vi "Event to CSV String PyExcel.vi"(8 "error in (no error)":errorcluster, 11 "Event":T1) -> (0 "error out":errorcluster, 2 "String":string)   [LabVIEW 2019, in "Logger.lvlib" / "Logger.lvclass"]
uses:
  Logger.lvclass
  Sensors/Detector/Event.ctl
  Sensors/Detector/Muon Detector.lvclass
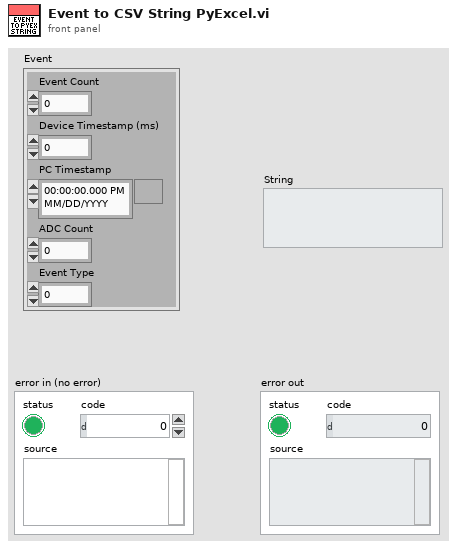
[diagram p1: front panel]
types:
  T1 = typedef "Muon Detector.lvclass/Event.ctl" = cluster{"Event Count":i32, "Device Timestamp (ms)":i32, "PC Timestamp":timestamp, "ADC Count":i32, "Event Type":u8}
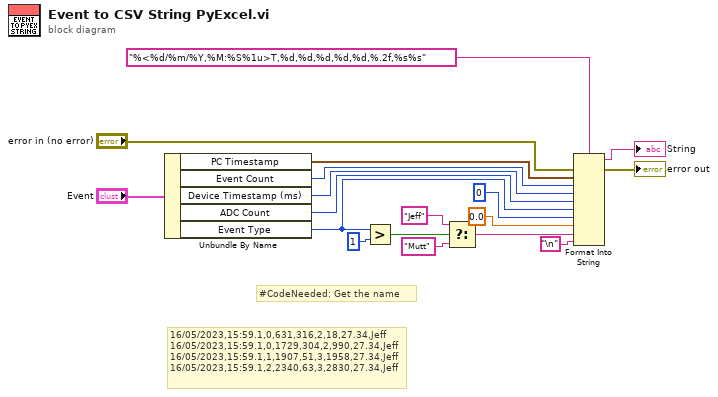
[diagram p0: block diagram]
diagram:
  # "16/05/2023,15:59.1,0,631,316,2,18,27.34,Jeff\n16/05/2023,15:59.1,0,1729,304,2,990,27.34,Jeff\n16/05/2023,15:59.1,1,1907,51,3,1958,27.34,Jeff\n16/05/2023,15:59.1,2,2340,63,3,2830,27.34,Jeff"
  # "#CodeNeeded: Get the name"
  n1 = Unbundle By Name("Event") -> ("PC Timestamp"=w1:timestamp, "Event Count"=w3:i32, "Device Timestamp (ms)"=w4:i32, "ADC Count"=w5:i32, "Event Type"=w7:u8)
  n2 = Greater?(x=w7, y=u8 1) -> (0:w9:bool)
  n3 = Select(t="Jeff", s=w9, f="Mutt") -> (s? t:f=w10:string)
  n4 = Format Into String(format string="%<%d/%m/%Y,%M:%S%1u>T,%d,%d,%d,%d,%d,%.2f,%s%s", error in="error in (no error)", w1, w3, w4, w5, w7, 0 ("input 6"), 0.0, w10, "\n") -> (resulting string=→"String":string, error out=→"error out":errorcluster)  [unwired: 1 in]
